vi "Close.vi"(8 "error in (no error)":errorcluster, 11 "Keysight 6700C in":refnum<class "Keysight 6700C.lvclass">) -> (0 "error out":errorcluster, 3 "Keysight 6700C out":refnum<class "Keysight 6700C.lvclass">)   [LabVIEW 2021, in "Concrete.lvlib" / "Keysight 6700C.lvclass"]
uses:
  Keysight 6700C.lvclass
  Keysight 6700C.lvclass/Keysight 6700C.ctl
  Harware Abstraction/AnalogIO/AIO.lvclass
  <instrlib>/Agilent N6700 Series/Agilent N6700 Series.lvlib
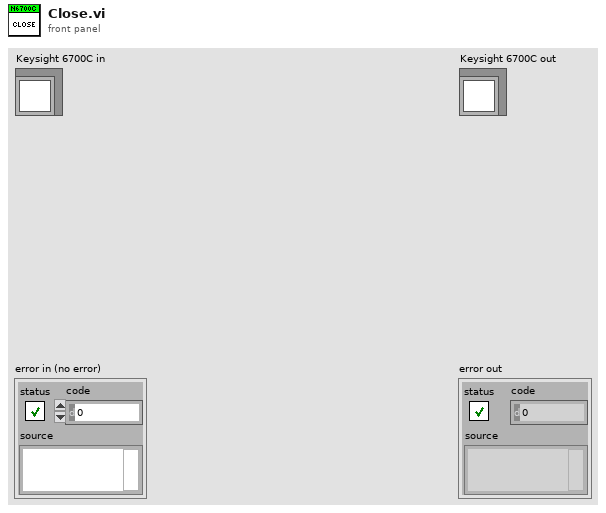
[diagram p1: front panel]
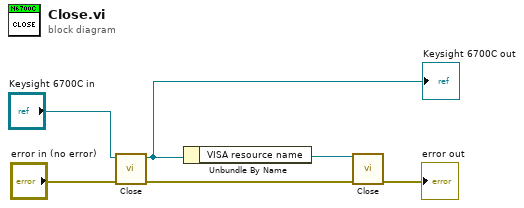
[diagram p0: block diagram]
diagram:
  n1 = call-parent <instrlib>:"Close.vi"("error in (no error)"="error in (no error)", "Instrument in"="Keysight 6700C in") -> ("error out"=w4:errorcluster, "Instrument out"=w2:refnum<class "Keysight 6700C.lvclass">)  [unwired: 8 in]
  "Keysight 6700C out" <- w2
  n2 = Unbundle By Name(w2) -> ("VISA resource name"=w1:refnum<visa-resource-name>)
  n3 = call <instrlib>:"Close.vi"("VISA resource name"=w1, "error in (no error)"=w4) -> ("error out"=→"error out":errorcluster)  [unwired: 13 in]
